vi "SrvPickEvent.vi"(0 "ref in":u64, 11 "error in (no error)":errorcluster) -> (4 "ref out":u64, 6 "return type":i32, 8 "Event":T1, 10 "EventReady":bool, 15 "error out":errorcluster)   [LabVIEW 2020, in "Snap7.lvlib"]
uses:
  Snap7.lvlib
  windows/lv_snap7.dll
panel:
  in  "var_Event":T1
  out "EvtReady":i32
  in  "var_EvtReady":i32
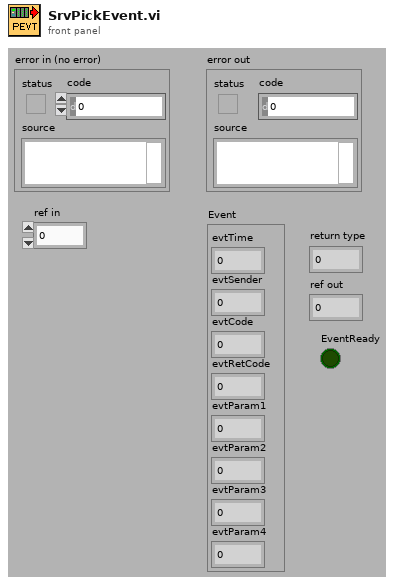
[diagram p1: front panel]
types:
  T1 = cluster{"evtTime":u32, "evtSender":i32, "evtCode":u32, "evtRetCode":u16, "evtParam1":u16, "evtParam2":u16, "evtParam3":u16, "evtParam4":u16}
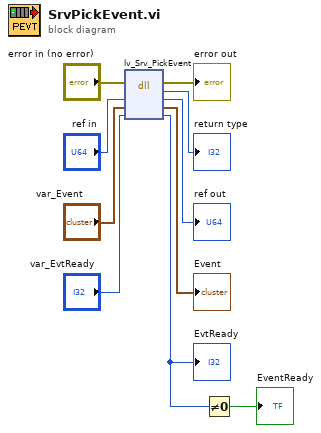
[diagram p0: block diagram]
diagram:
  n1 = dll-call lib="PTH2iabs CUsersFeng项目HLCEPS300-1老性能试验台SourcesSnap7libwindowslv_snap7.dll" fn="lv_Srv_PickEvent"(error in="error in (no error)", "Server"="ref in", "Event"="var_Event", "EvtReady"="var_EvtReady") -> (error out=→"error out":errorcluster, "return type"=→"return type":i32, "Server"=→"ref out":u64, "Event"=→"Event":T1, "EvtReady"=w4:i32)  [unwired: 2 in, 1 out]
  "EvtReady" <- w4
  n2 = Not Equal To 0?(x=w4) -> (x != 0?=→"EventReady":bool)
